vi "MS SQL_Read_TS_Data.vi"(8 "error in (no error)":errorcluster, 10 "Enable?":bool=TRUE, 11 "Ref in":T3={"MS SQL Connection"=refnum, "UDL File"=path "", "Time"="", "DCODE"="", "WIP+1"=0, "MC No?"=0, "POKAYOKE?"=FALSE, "Expected Result"="", "Result [Status]"="", "Clock"=0.0, "RFID"="", "WIP Queue"=refnum, "TS Parameter"={"ProfitCenterCode"="", "LineCode"="", "WorkOrderNumber"="", "Model"="", "Model_with_Prefix"="", "VendorCode"="", "SetParameterDateCode"="", "PokaYoke"=0, "Target"=1, "Live_DateCode"="", "CustomerPartNumber"="", "Hand"="", "sBarcode"=FALSE, "FCA"=0, "Ent_Stamp"=timestamp(0 s since 1904-01-01), "STS_CD"=0.0}, "Data_Queue"=[], "RFID Serial No."=""} {"TS Parameter"."FCA" format="%01d"; "TS Parameter"."Target" min=1 max=100000; "TS Parameter"."PokaYoke" min=0 max=1}) -> (0 "error out":errorcluster, 1 "TS Parameter":T2={"ProfitCenterCode"="", "LineCode"="", "WorkOrderNumber"="", "Model"="", "Model_with_Prefix"="", "VendorCode"="", "SetParameterDateCode"="", "PokaYoke"=0, "Target"=1, "Live_DateCode"="", "CustomerPartNumber"="", "Hand"="", "sBarcode"=FALSE, "FCA"=0, "Ent_Stamp"=timestamp(0 s since 1904-01-01), "STS_CD"=0.0} {"FCA" format="%01d"; "Target" min=1 max=100000; "PokaYoke" min=0 max=1}, 2 "Set Parameter Ok?":bool, 3 "Ref Out":T3={"MS SQL Connection"=refnum, "UDL File"=path "", "Time"="", "DCODE"="", "WIP+1"=0, "MC No?"=0, "POKAYOKE?"=FALSE, "Expected Result"="", "Result [Status]"="", "Clock"=0.0, "RFID"="", "WIP Queue"=refnum, "TS Parameter"={"ProfitCenterCode"="", "LineCode"="", "WorkOrderNumber"="", "Model"="", "Model_with_Prefix"="", "VendorCode"="", "SetParameterDateCode"="", "PokaYoke"=0, "Target"=1, "Live_DateCode"="", "CustomerPartNumber"="", "Hand"="", "sBarcode"=FALSE, "FCA"=0, "Ent_Stamp"=timestamp(0 s since 1904-01-01), "STS_CD"=0.0}, "Data_Queue"=[], "RFID Serial No."=""} {"TS Parameter"."FCA" format="%01d"; "TS Parameter"."Target" min=1 max=100000; "TS Parameter"."PokaYoke" min=0 max=1}, 4 "Target?":bool, 5 "RFID Count":i32 format="%02d", 6 "RFID Serial No":string, 7 "Pokeyoke?":bool)   [LabVIEW 2020]
uses:
  Controls/TD SQL.ctl
  <vilib>/addons/database/Connection.llb/Conn ObjectReference.ctl
  Controls/WIP_State.ctl
  Controls/TS_Parameter.ctl
  Controls/Disp_Parameter.ctl
  MS_Global.vi
  <vilib>/addons/database/NI_Database_API.lvlib
panel:
  out "Disp. Parameter":T1
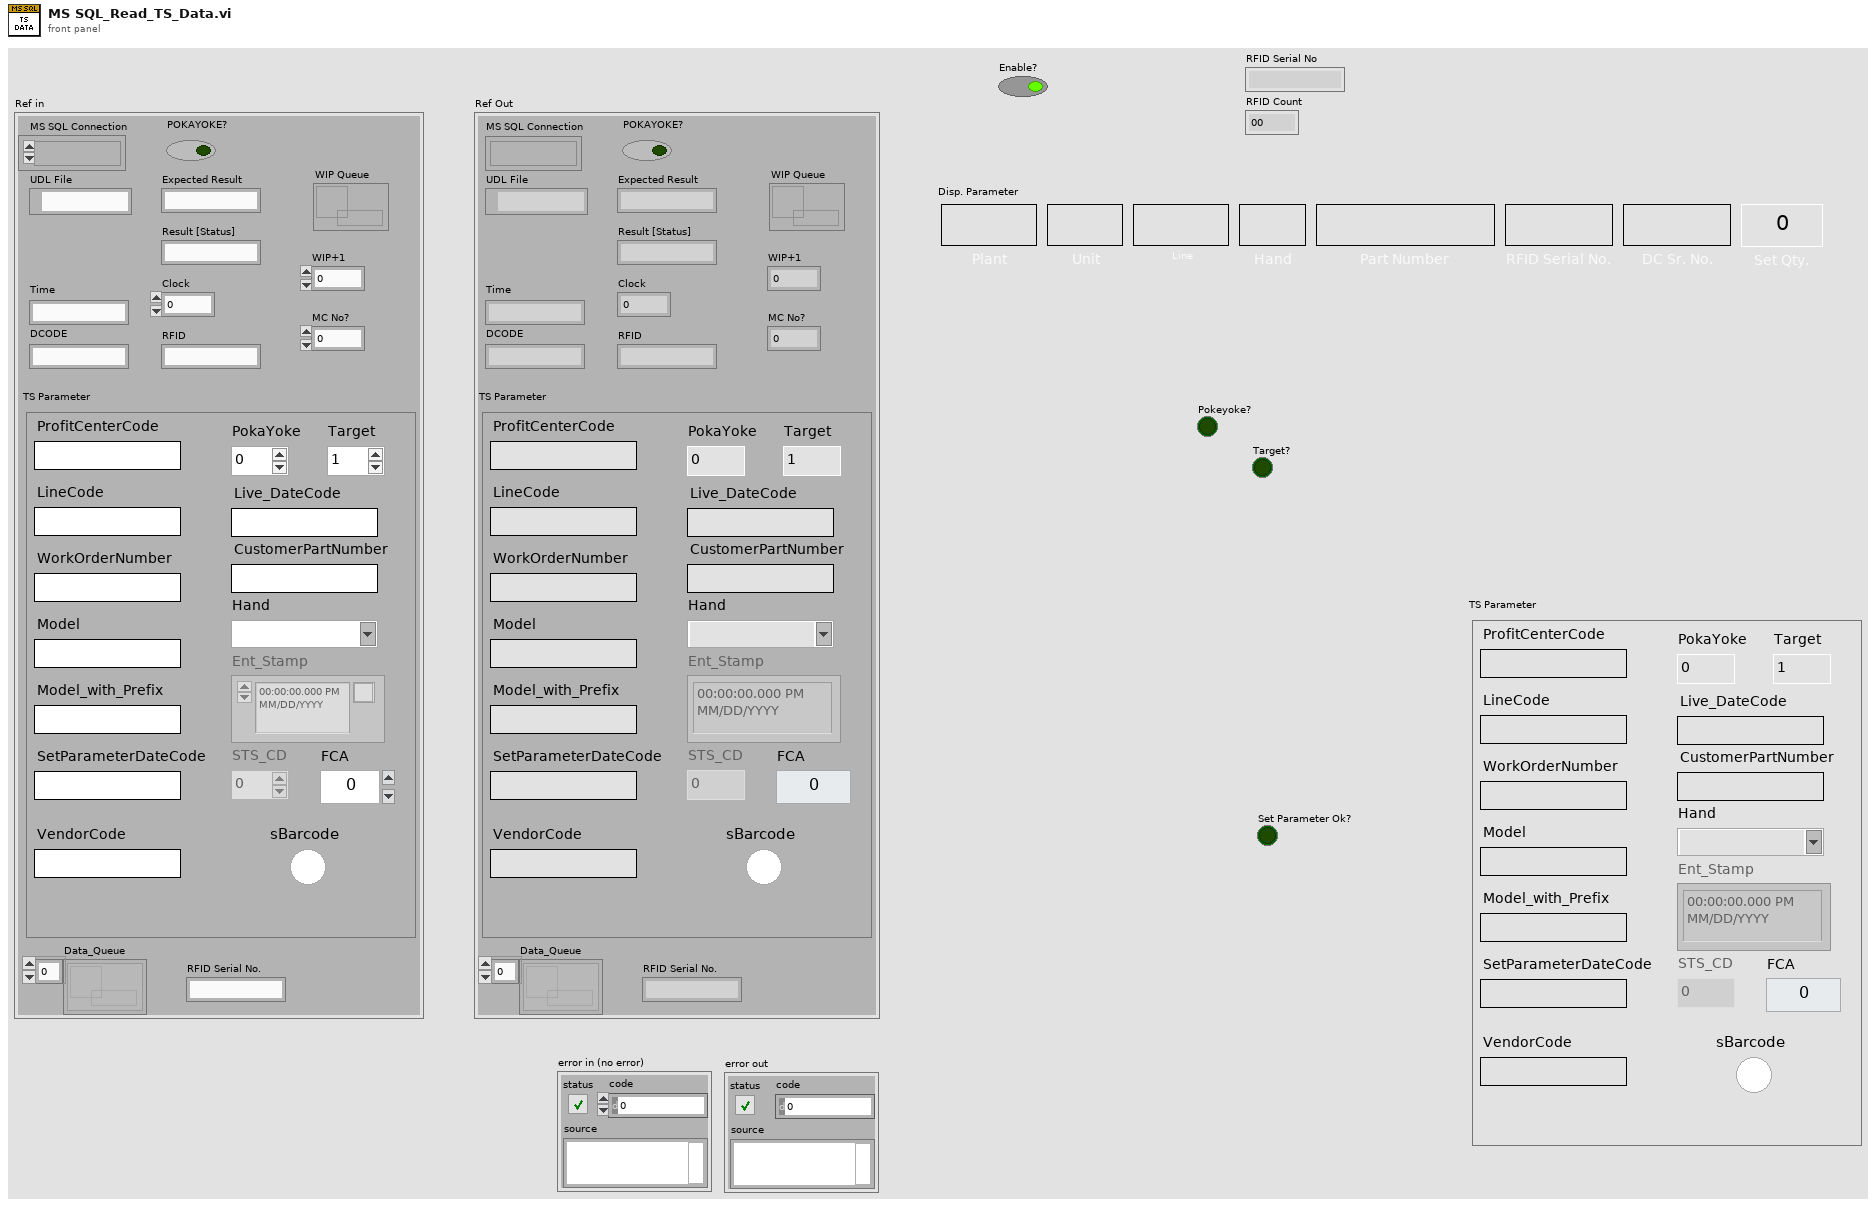
[diagram p1: front panel]
types:
  T1 = typedef "Disp_Parameter.ctl" = cluster{"Plant":string, "Unit":string, "Line":string, "Hand":string, "Part Number":string, "RFID Serial No.":string, "DC Sr. No.":string, "Set Qty.":i32}
  T2 = typedef "TS_Parameter.ctl" = cluster{"ProfitCenterCode":string, "LineCode":string, "WorkOrderNumber":string, "Model":string, "Model_with_Prefix":string, "VendorCode":string, "SetParameterDateCode":string, "PokaYoke":i32, "Target":i32, "Live_DateCode":string, "CustomerPartNumber":string, "Hand":string, "sBarcode":bool, "FCA":i32, "Ent_Stamp":timestamp, "STS_CD":dbl}
  T3 = typedef "TD SQL.ctl" = cluster{"MS SQL Connection":T4, "UDL File":path, "Time":string, "DCODE":string, "WIP+1":i64, "MC No?":i32, "POKAYOKE?":bool, "Expected Result":string, "Result [Status]":string, "Clock":dbl, "RFID":string, "WIP Queue":refnum<queue>, "TS Parameter":T2, "Data_Queue":refnum<queue>[], "RFID Serial No.":string}
  T4 = typedef "NI_Database_API.lvlib/Conn ObjectReference.ctl" = refnum<k1>
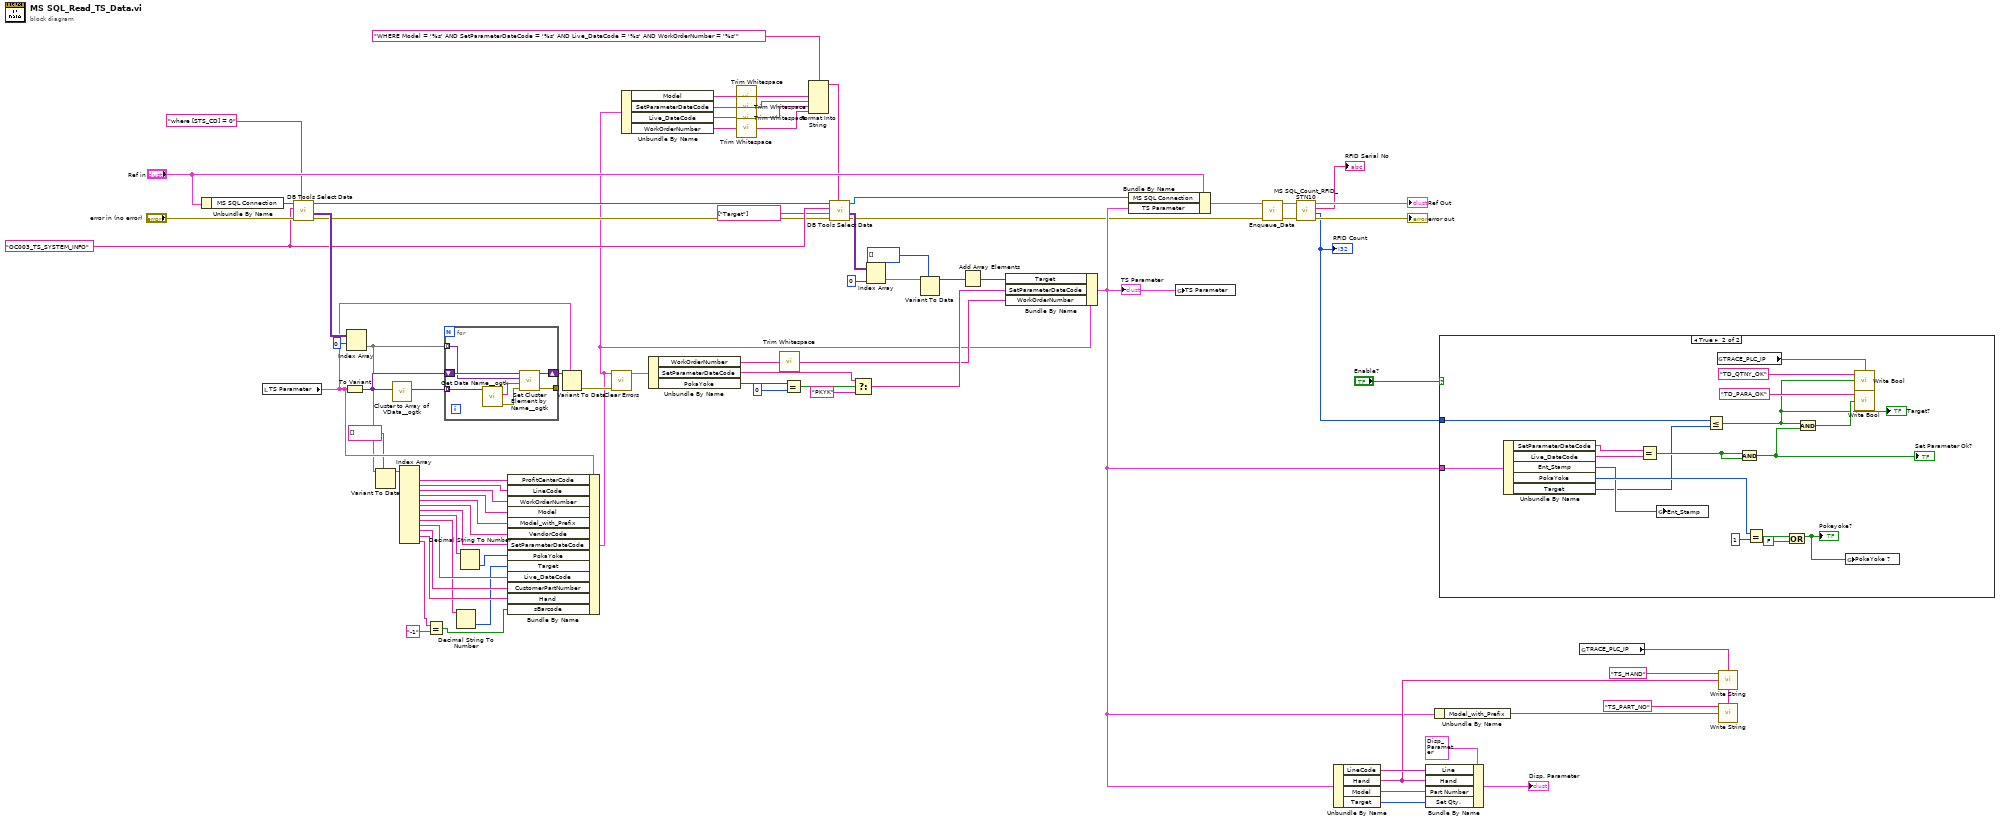
[diagram p0: block diagram]
diagram:
  w65 = "OC003_TS_SYSTEM_INFO"
  n1 = Unbundle By Name("Ref in") -> ("MS SQL Connection"=w79:T4)
  n2 = local read "TS Parameter"() -> (w22:T2)
  n3 = call <vilib>:"DB Tools Select Data.vi"("condition"="where [STS_CD] = 0", "error in (no error)"="error in (no error)", "table"=w65, "connection reference"=w79) -> ("error out"=w63:errorcluster, "data"=w73:variant[][], "connection reference out"=w67:T4)  [unwired: 2 in]
  n4 = To Variant(anything=w22) -> (Variant=w75:variant)
  n5 = Index Array(array=w73, index (row)=0) -> (element=w21:variant[])  [unwired: 1 in]
  n6 = Variant To Data(type=string[] [], Variant=w21) -> (data=w19:string[])  [unwired: 1 in, 1 out]
  n7 = call <userlib>:"Cluster to Array of VData__ogtk.vi"("Cluster"=w75) -> ("Array of VData"=w76:variant[])  [unwired: 9 in, 1 out]
  n8 = Index Array(array=w19) -> (element #1=w18:string, element #2=w16:string, element #3=w15:string, element #4=w14:string, element #5=w13:string, element #6=w12:string, element #7=w11:string, element #8=w7:string, element #9=w5:string, element #10=w10:string, element #11=w9:string, element #12=w8:string, element #13=w3:string)  [unwired: 13 in]
  n9 = Equal?(x=w3, y="-1") -> (x = y?=w1:bool)
  n10 = for {
    tunnel: w21 -> [w84] mode=indexing
    tunnel: w76 -> [w88] mode=indexing
    shift-right: [w86] -> w74
    shift-left: w75 -> [w87]
    tunnel: [w83] -> _
    n11 = call <userlib>:"Get Data Name__ogtk.vi"("Data"=w88) -> ("error out"=w82:errorcluster, "Data Name"=w85:string)  [unwired: 8 in, 1 out]
    n12 = call <userlib>:"Set Cluster Element by Name__ogtk.vi"("error in (no error)"=w82, "Element Name (\"\": New Element Data Name)"=w85, "New Element Value"=w84, "Cluster"=w87) -> ("error out"=w83:errorcluster, "VCluster out"=w86:variant)  [unwired: 5 in, 1 out]
  }
  n13 = Decimal String To Number(string=w5) -> (number=w4:i32)  [unwired: 2 in, 1 out]
  n14 = Decimal String To Number(string=w7) -> (number=w6:i32)  [unwired: 2 in, 1 out]
  n15 = Bundle By Name(cluster=w22, "ProfitCenterCode"=w18, "LineCode"=w16, "WorkOrderNumber"=w15, "Model"=w14, "Model_with_Prefix"=w13, "VendorCode"=w12, "SetParameterDateCode"=w11, "PokaYoke"=w6, "Target"=w4, "Live_DateCode"=w10, "CustomerPartNumber"=w9, "Hand"=w8, "sBarcode"=w1) -> (w17:T2)
  n16 = Variant To Data(type=w22, Variant=w74) -> (error out=w72:errorcluster)  [unwired: 1 in, 1 out]
  n17 = call <vilib>:"Clear Errors.vi"("error in (no error)"=w72) -> ()  [unwired: 5 in, 2 out]
  n18 = Unbundle By Name(w17) -> ("Model"=w71:string, "SetParameterDateCode"=w70:string, "Live_DateCode"=w69:string, "WorkOrderNumber"=w58:string)
  n19 = Unbundle By Name(w17) -> ("WorkOrderNumber"=w37:string, "SetParameterDateCode"=w39:string, "PokaYoke"=w36:i32)
  n20 = call <vilib>:"Trim Whitespace.vi"("string"=w71) -> ("trimmed string"=w52:string)  [unwired: 1 in]
  n21 = call <vilib>:"Trim Whitespace.vi"("string"=w70) -> ("trimmed string"=w53:string)  [unwired: 1 in]
  n22 = call <vilib>:"Trim Whitespace.vi"("string"=w69) -> ("trimmed string"=w54:string)  [unwired: 1 in]
  n23 = call <vilib>:"Trim Whitespace.vi"("string"=w58) -> ("trimmed string"=w55:string)  [unwired: 1 in]
  n24 = call <vilib>:"Trim Whitespace.vi"("string"=w37) -> ("trimmed string"=w32:string)  [unwired: 1 in]
  n25 = Equal?(x=w36, y=0) -> (x = y?=w35:bool)
  n26 = Format Into String(format string="WHERE Model = '%s' AND SetParameterDateCode = '%s' AND Live_DateCode = '%s' AND WorkOrderNumber = '%s'" ("ProfitCenterCode"), w52, w53, w54, w55) -> (resulting string=w62:string)  [unwired: 2 in, 1 out]
  n27 = call <vilib>:"DB Tools Select Data.vi"("condition"=w62, "error in (no error)"=w63, "columns"=string[] ["Target"], "table"=w65, "connection reference"=w67) -> ("error out"=w29:errorcluster, "data"=w61:variant[][], "connection reference out"=w66:T4)  [unwired: 1 in]
  n28 = Select(t=w39, s=w35, f="PKYK") -> (s? t:f=w33:string)
  n29 = Index Array(array=w61, index (col)=0 ("index (row)")) -> (element=w60:variant[])  [unwired: 1 in]
  n30 = Variant To Data(type=i32[] [], Variant=w60) -> (data=w57:i32[])  [unwired: 1 in, 1 out]
  n31 = Add Array Elements(numeric array=w57) -> (sum=w56:i32)
  n32 = Bundle By Name(cluster=w17, "Target"=w56, "SetParameterDateCode"=w33, "WorkOrderNumber"=w32) -> (w31:T2)
  "TS Parameter" <- w31
  n33 = Bundle By Name(cluster="Ref in", "MS SQL Connection"=w66, "TS Parameter"=w31) -> (w30:T3)
  n34 = global write "MS_Global.vi" "TS Parameter"(w31) -> ()
  n35 = call "Enqueue_Data.vi"("error in (no error)"=w29, "Ref in"=w30) -> ("error out"=w26:errorcluster, "Ref out"=w28:T3)  [unwired: 8 in]
  n36 = call "MS SQL_Count_RFID_STN10.vi"("error in (no error)"=w26, "Ref in"=w28) -> ("error out"=→"error out":errorcluster, "Count"=w23:i32, "Count[s]"=→"RFID Serial No":string, "Ref Out"=→"Ref Out":T3)  [unwired: 5 in, 1 out]
  "RFID Count" <- w23
  n37 = Unbundle By Name(w31) -> ("LineCode"=w47:string, "Hand"=w43:string, "Model"=w46:string, "Target"=w45:i32)
  n38 = Bundle By Name(cluster=T1 {"Plant"="BD02", "Unit"="U64", "Line"="C10", "Hand"="RH", "Part Number"="29032639", "RFID Serial No."="000001", "DC Sr. No."="000001", "Set Qty."=7200} ("Parameter"), "Line"=w47, "Hand"=w43, "Part Number"=w46, "Set Qty."=w45) -> (→"Disp. Parameter":T1)
  n39 = Unbundle By Name(w31) -> ("Model_with_Prefix"=w40:string)
  n40 = case shown="True" "Enable?" {
    tunnel: w31 -> [_ w93]
    tunnel: w23 -> [_ w89]
    frame False {
    }
    frame True {
      n41 = Unbundle By Name(w93) -> ("SetParameterDateCode"=w106:string, "Live_DateCode"=w105:string, "Ent_Stamp"=w101:timestamp, "PokaYoke"=w104:i32, "Target"=w92:i32)
      n42 = Equal?(x=w106, y=w105) -> (x = y?=w98:bool)
      n43 = global write "MS_Global.vi" "Ent_Stamp"(w101) -> ()
      n44 = Less Or Equal?(x=w89, y=w92) -> (x <= y?=w96:bool)
      "Target?" <- w96
      n45 = global read "MS_Global.vi" "TRACE_PLC_IP"() -> (w95:string)
      n46 = Compound Arithmetic op=AND(w98, w98) -> (w94:bool)
      "Set Parameter Ok?" <- w94
      n47 = Equal?(x=w104, y=1) -> (x = y?=w102:bool)
      n48 = Compound Arithmetic op=OR(w102, FALSE ("value")) -> (w90:bool)
      "Pokeyoke?" <- w90
      n49 = Compound Arithmetic op=AND(w96, w94) -> (w97:bool)
      n50 = global write "MS_Global.vi" "PokaYoke ?"(w90) -> ()
      n51 = call "Write Bool.vi"("Network Path"=w95, "Int"=w96, "Tag Name"="TD_QTNY_OK" ("Network Path")) -> ()  [unwired: 2 in]
      n52 = call "Write Bool.vi"("Network Path"=w95, "Int"=w97, "Tag Name"="TD_PARA_OK" ("Network Path")) -> ()  [unwired: 2 in]
    }
  }
  n53 = global read "MS_Global.vi" "TRACE_PLC_IP"() -> (w42:string)
  n54 = call "Write String.vi"("Network Path"=w42, "String"=w43, "Tag Name"="TS_HAND") -> ()  [unwired: 2 in]
  n55 = call "Write String.vi"("Network Path"=w42, "String"=w40, "Tag Name"="TS_PART_NO") -> ()  [unwired: 2 in]
